vi "Fast AutoFocus.vi"(6 "Speed(mm/s)":dbl=0.5, 7 "Start Z":dbl, 8 "error in":errorcluster, 9 "Range(mm)":dbl=0.02, 10 "Steps":i32=10, 11 "CameraTool In":refnum<class "CameraTool Class.lvclass">) -> (0 "error out":errorcluster, 2 "focus height":dbl, 3 "CameraTool Out":refnum<class "CameraTool Class.lvclass">)   [LabVIEW 2017, in "CameraTool Class.lvclass"]
doc: "This VI returns the \"variance of laplacians\" measure of image focus."
uses:
  CameraTool Class.lvclass
  gVision API/gVision/gVision.lvlib
  Vec3d Class/Vec3d Class.lvclass
  Config Manager Class/Type Definitions/Camera Enum.ctl
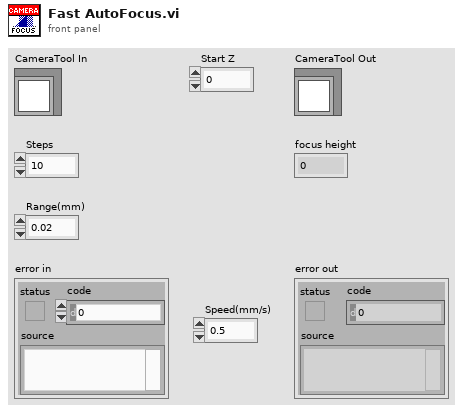
[diagram p1: front panel]
types:
  T1 = typedef "Camera Enum.ctl" = enum16{"gantryhead", "NEEDLE CALIBRATION X", "NEEDLE CALIBRATION Y", "STAND CAMERA", "SIMRAN WEBCAM"}
  T2 = typedef "IMAQ Image.ctl" = refnum<image>
  T3 = typedef "Physical Image.ctl" = cluster{"Image Position":refnum<class "Vec3d Class.lvclass">, "Image Reference":T2, "Field of View":cluster{"x(mm)":dbl, "y(mm)":dbl}}
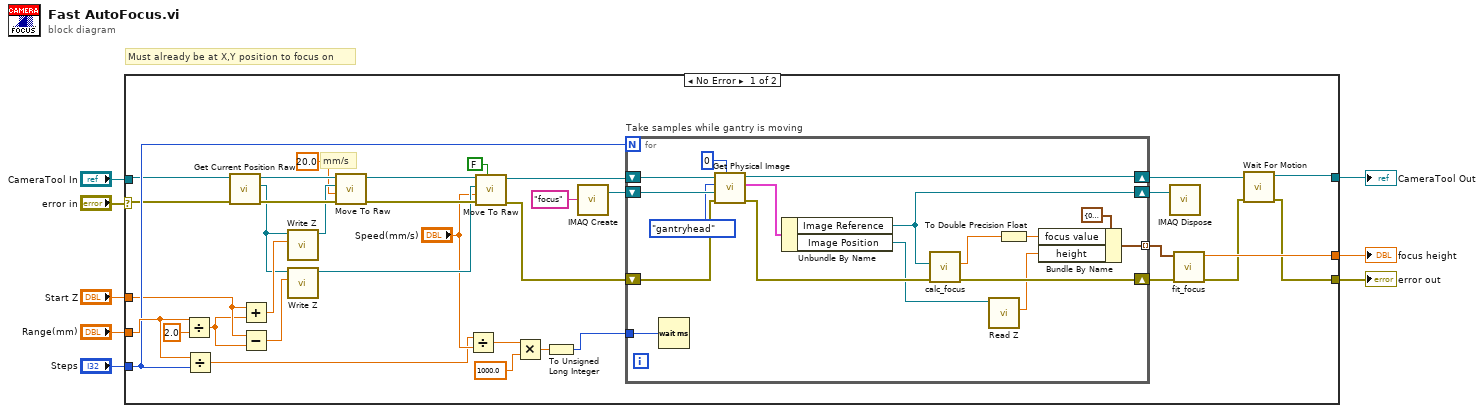
[diagram p0: block diagram]
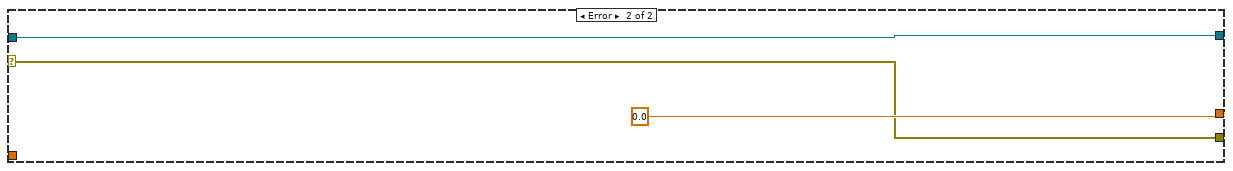
[diagram p2: hidden frame]
diagram:
  # "Must already be at X,Y position to focus on"
  n1 = case shown="No Error" "error in" {
    selector: "error in" -> [w33 w62]
    tunnel: "Start Z" -> [w26 _]
    tunnel: "CameraTool In" -> [w34 w64]
    tunnel: [w43 sgl 0.0 ("return type")] -> w5
    tunnel: [w9 w62] -> w4
    tunnel: [w11 w64] -> w3
    tunnel: "Steps" -> [w40 _]
    tunnel: "Range(mm)" -> [w41 _]
    frame No Error {
      # "mm/s"
      n2 = Divide(x=w41, y=2.0) -> (x/y=w25:dbl)
      n3 = Divide(x=w41, y=w40) -> (x/y=w18:dbl)
      n4 = call-dynamic "Get Current Position Raw.vi"("error in"=w33, "Gantry in"=w34) -> ("error out"=w35:errorcluster, "Vec3d Class out"=w27:refnum<class "Vec3d Class.lvclass">, "Gantry out"=w36:refnum<class "CameraTool Class.lvclass">)  [unwired: 7 in]
      n5 = Add(x=w26, y=w25) -> (x+y=w32:dbl)
      n6 = Subtract(x=w26, y=w25) -> (x-y=w24:dbl)
      n7 = call-dynamic "Write Z.vi"("Z"=w32, "Vec3d Class in"=w27) -> ("Vec3d Class out"=w31:refnum<class "Vec3d Class.lvclass">)  [unwired: 8 in, 1 out]
      n8 = call-dynamic "Write Z.vi"("Z"=w24, "Vec3d Class in"=w27) -> ("Vec3d Class out"=w23:refnum<class "Vec3d Class.lvclass">)  [unwired: 8 in, 1 out]
      n9 = call-dynamic "Move To Raw.vi"("error in"=w35, "Speed"=20.0, "Destination"=w31, "Gantry in"=w36) -> ("error out"=w28:errorcluster, "Gantry out"=w29:refnum<class "CameraTool Class.lvclass">)  [unwired: 6 in]
      n10 = Divide(x=w18, y="Speed(mm/s)") -> (x/y=w17:dbl)
      n11 = call-dynamic "Move To Raw.vi"("Wait?"=FALSE, "error in"=w28, "Speed"="Speed(mm/s)", "Destination"=w23, "Gantry in"=w29) -> ("error out"=w20:errorcluster, "Gantry out"=w21:refnum<class "CameraTool Class.lvclass">)  [unwired: 5 in]
      n12 = Multiply(x=w17, y=1000.0) -> (x*y=w15:dbl)
      n13 = To Unsigned Long Integer(number=w15) -> (unsigned 32bit integer=w14:u32)
      n14 = call "IMAQ Create"("Image Name"="focus") -> ("New Image"=w38:T2)  [unwired: 4 in, 1 out]
      n15 = for "Take samples while gantry is moving" {
        N: w40 -> [_]
        shift-right: [w61] -> w12
        shift-left: w21 -> [w57]
        shift-right: [w60] -> w44
        shift-left: w20 -> [w52]
        shift-right: [w54] -> w37
        shift-left: w38 -> [w59]
        tunnel: w14 -> [w56]
        tunnel: [w47] -> w13 mode=indexing
        n16 = Wait (ms)(milliseconds to wait=w56) -> ()  [unwired: 1 out]
        n17 = call-dynamic "Get Physical Image.vi"("Delay(milliseconds)"=0, "error in"=w52, "Image In"=w59, "Camera Name"=Camera_Enum."gantryhead", "Gantry in"=w57) -> ("error out"=w58:errorcluster, "Physical Image"=w55:T3, "Gantry out"=w61:refnum<class "CameraTool Class.lvclass">)  [unwired: 4 in]
        n18 = Unbundle By Name(w55) -> ("Image Reference"=w54:T2, "Image Position"=w53:refnum<class "Vec3d Class.lvclass">)
        n19 = call "calc_focus.vi"("error in"=w58, "Image"=w54) -> ("error out"=w60:errorcluster, "focus"=w50:sgl)  [unwired: 7 in, 1 out]
        n20 = call-dynamic "Read Z.vi"("Vec3d Class in"=w53) -> ("Z"=w48:dbl)  [unwired: 8 in, 2 out]
        n21 = To Double Precision Float(number=w50) -> (double precision float=w49:dbl)
        n22 = Bundle By Name(cluster=cluster{"focus value":dbl, "height":dbl} {"focus value"=0.0, "height"=0.0} ("Focus Measurement"), "focus value"=w49, "height"=w48) -> (w47:cluster{"focus value":dbl, "height":dbl})
      }
      n23 = call "IMAQ Dispose"("Image"=w37) -> ()  [unwired: 5 in, 1 out]
      n24 = call "fit_focus.vi"("error in"=w44, "Focus Measurements"=w13) -> ("error out"=w10:errorcluster, "focus height"=w43:dbl)  [unwired: 7 in, 1 out]
      n25 = call-dynamic "Wait For Motion.vi"("error in"=w10, "Gantry in"=w12) -> ("error out"=w9:errorcluster, "Gantry out"=w11:refnum<class "CameraTool Class.lvclass">)  [unwired: 8 in]
    }
    frame Error {
    }
  }
  "CameraTool Out" <- w3
  "error out" <- w4
  "focus height" <- w5
